vi "FindServo_NoWhile.vi"(0 "Amplitude Reference Array":refnum<vi>[](array[refnum]), 1 "Parameter Reference Arrary":refnum<vi>[](array[refnum]), 7 "Parameter Cluster":T1={"Αmplitude (Deg)"=0.0, "Amplitude (cm)"=4.0, "Frequency (Hz)"=1.0, "Number of Waves"=1.0, "Length of Segments (cm)"=10.0, "Wave Exponential"=2.0, "Number of Servos"=5.0, "Bend Amplitude 1"=0.1, "Bend Amplitude 2"=0.2, "Bend Phase 1"=0.0, "Bend Phase 2"=0.8499}, 8 "Wave Form":u16(ring) items=["Sine", "Exponentional Sine", "Two Beam Bending", "Flat Plate"], 12 "Wind Up":bool, 13 "Start Time (Tick Count-millis)":u32, 14 "Wind Down":bool, 15 "Wind Down Time":i32=5, 16 "Stop In":bool, 17 "Stop Pressed Shift In (False)":bool, 19 "Ms Since Stop Shift In (Start Time)":u32, 23 "Stop In Reference":refnum<vi>, 27 "S since stop Shift In":dbl) -> (18 "Stop Out":bool, 20 "phi":dbl[](array[numeric]), 21 "X Nodes":dbl[](array[numeric]), 22 "Y Nodes":dbl[](array[numeric]), 24 "Stop Pressed Shift Out (False)":bool, 25 "MS Since Stop Shift Out":u32, 26 "S since stop Shift Out":dbl)   [LabVIEW 2017]
panel:
  out "Simulation Time":dbl
  # "Off"
  # "On"
  # "Off"
  # "On"
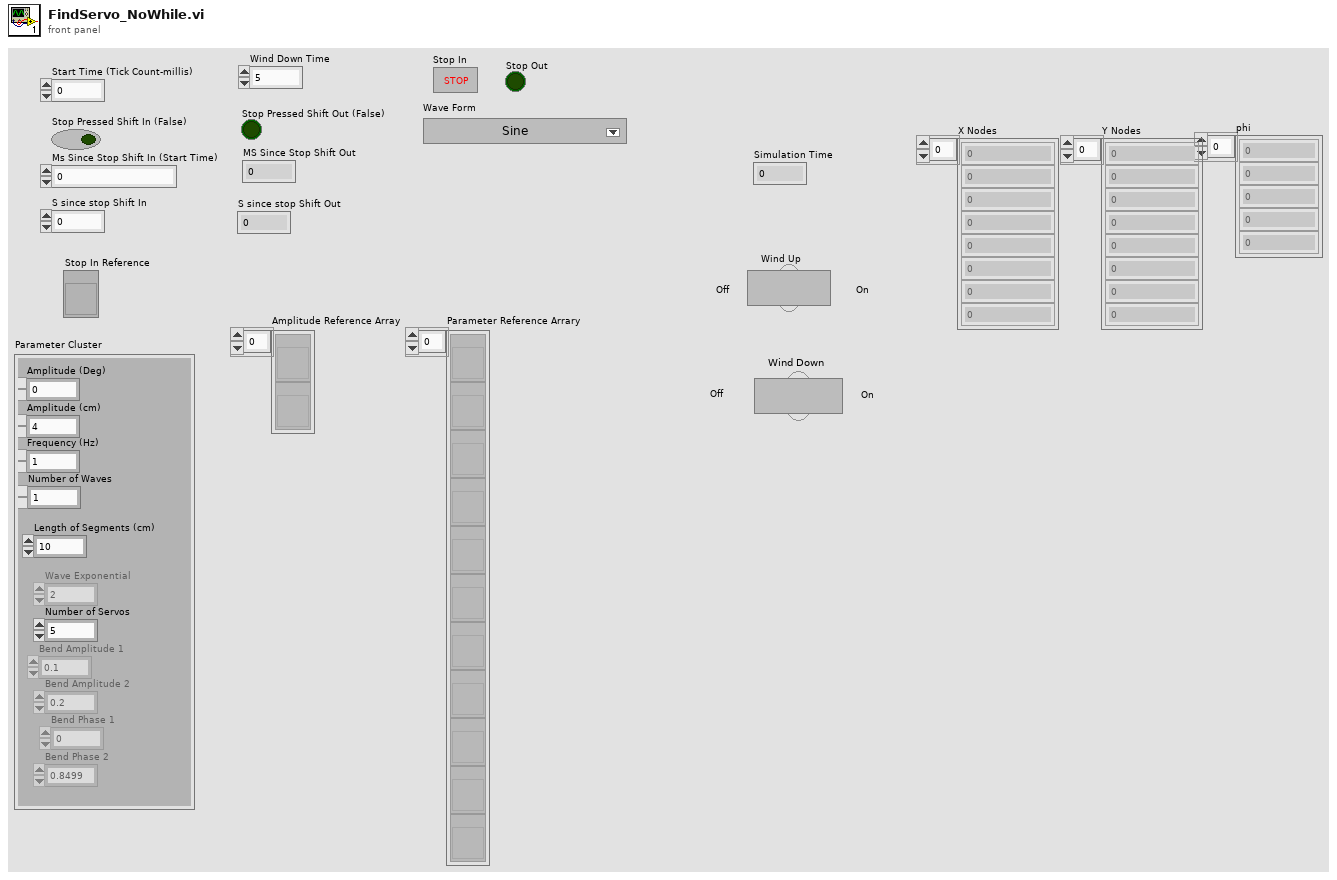
[diagram p1: front panel]
types:
  T1 = cluster{"Αmplitude (Deg)":dbl, "Amplitude (cm)":dbl, "Frequency (Hz)":dbl, "Number of Waves":dbl, "Length of Segments (cm)":dbl, "Wave Exponential":dbl, "Number of Servos":dbl, "Bend Amplitude 1":dbl, "Bend Amplitude 2":dbl, "Bend Phase 1":dbl, "Bend Phase 2":dbl}
  T2 = enum8{"Enabled", "Disabled", "Disabled and Grayed Out"}
  T3 = enum8{"Enabled", "Disabled", "Disabled and Grayed Out"}[]
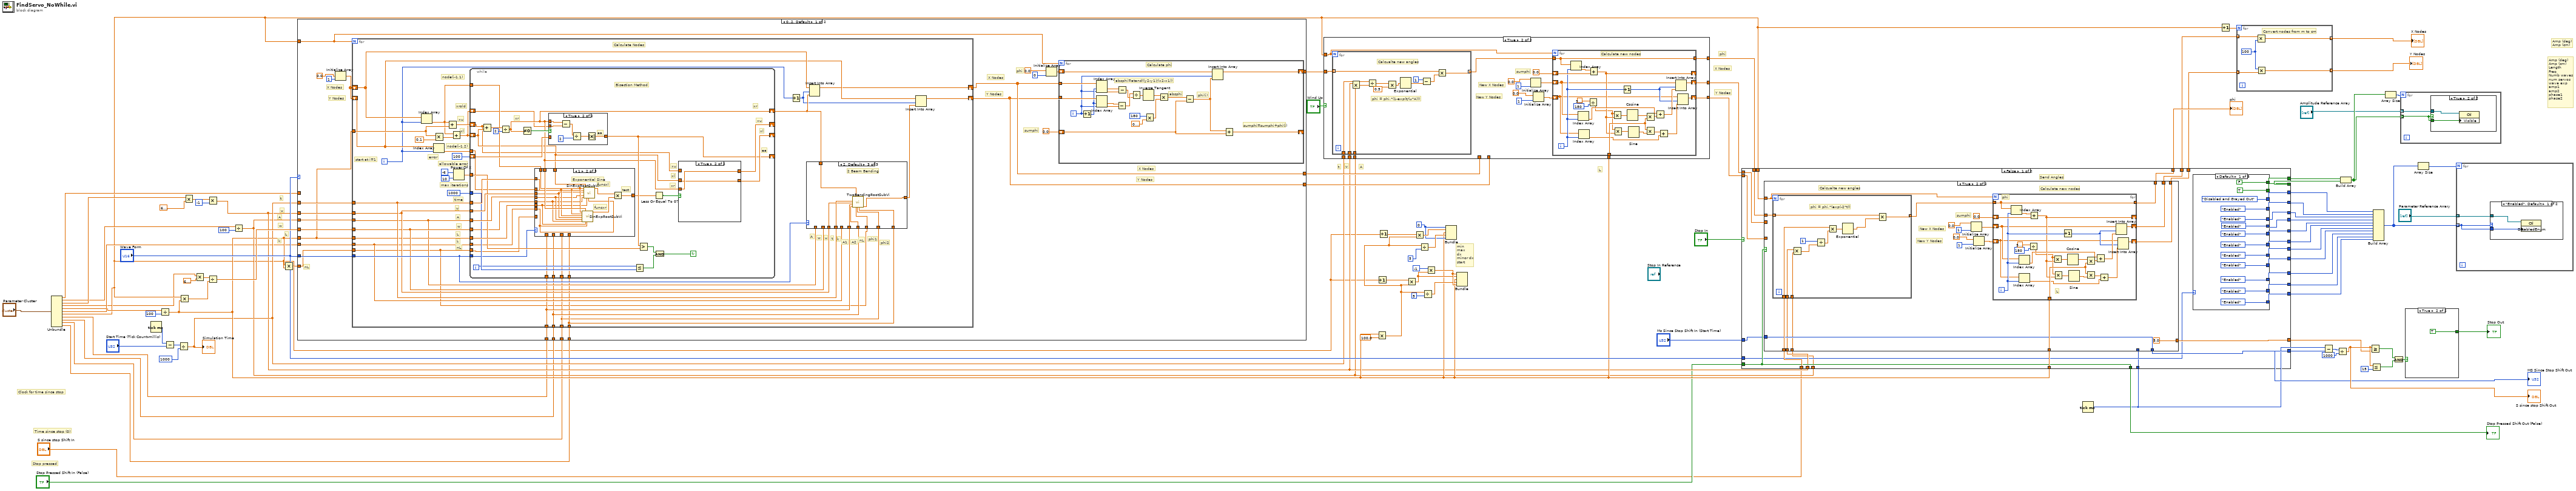
[diagram p0: block diagram]
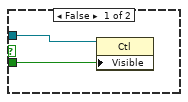
[diagram p2: hidden frame]
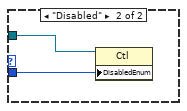
[diagram p3: hidden frame]
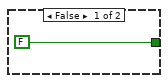
[diagram p4: hidden frame]
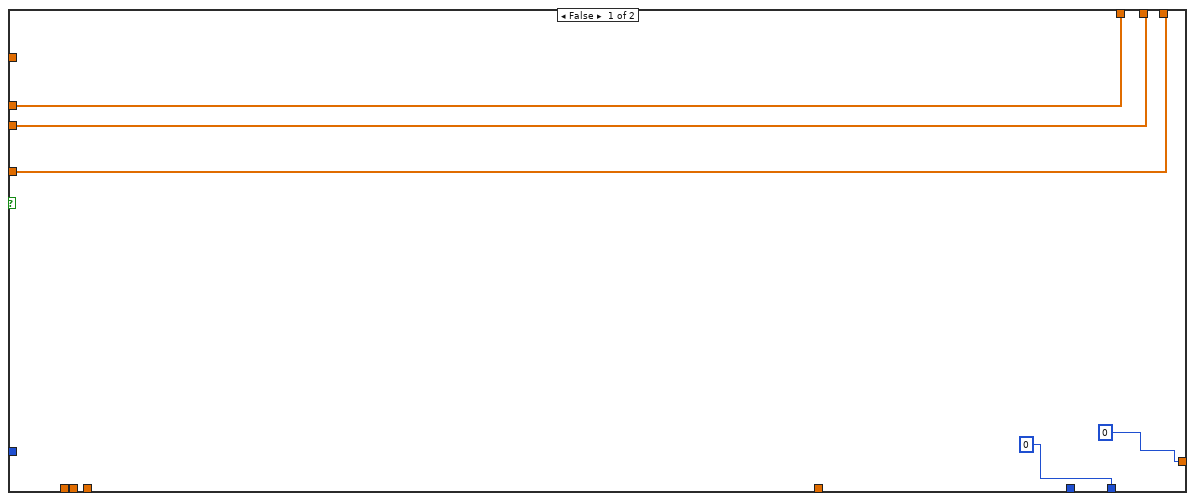
[diagram p5: hidden frame]
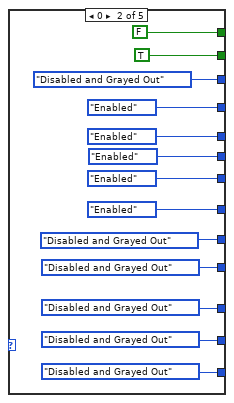
[diagram p6: hidden frame]
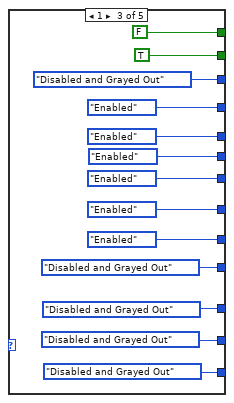
[diagram p7: hidden frame]
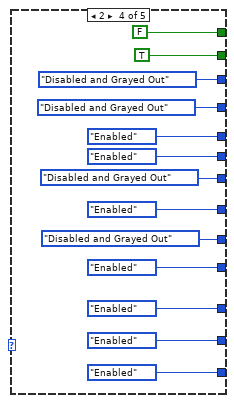
[diagram p8: hidden frame]
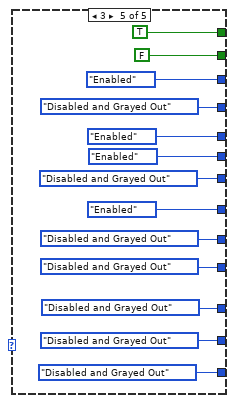
[diagram p9: hidden frame]
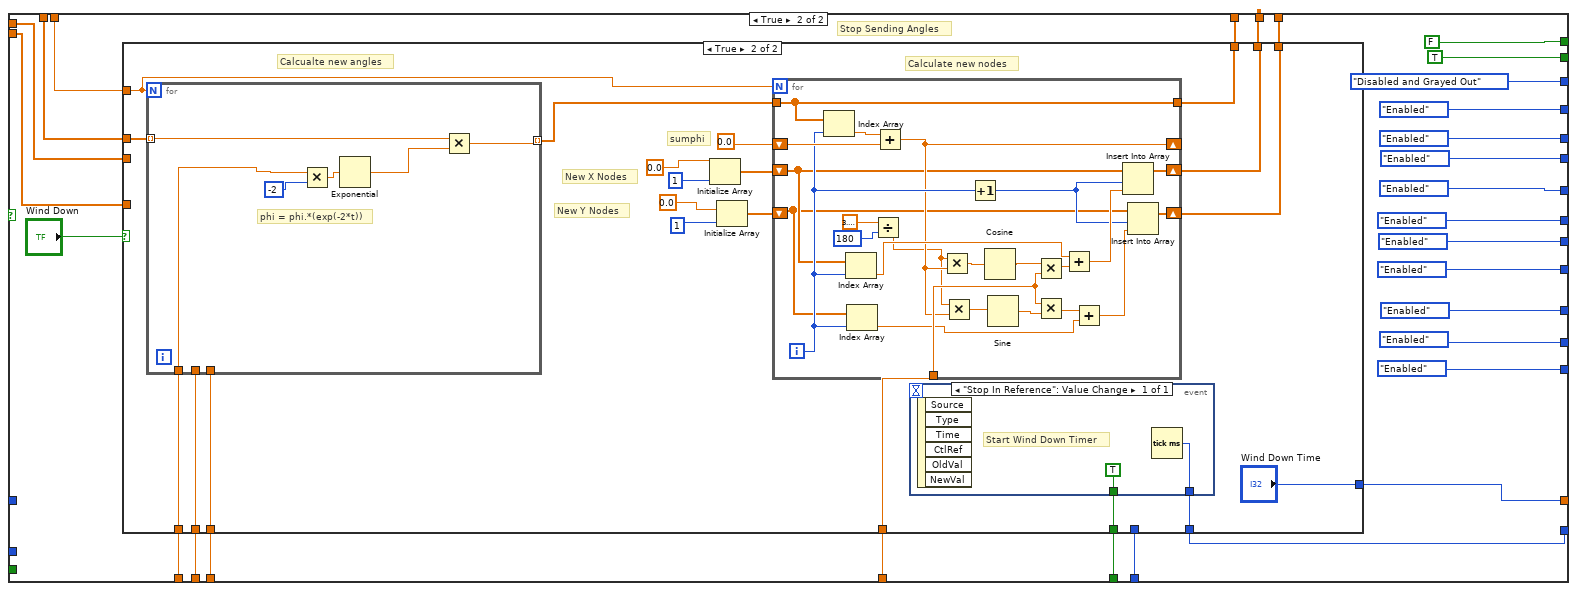
[diagram p10: hidden frame]
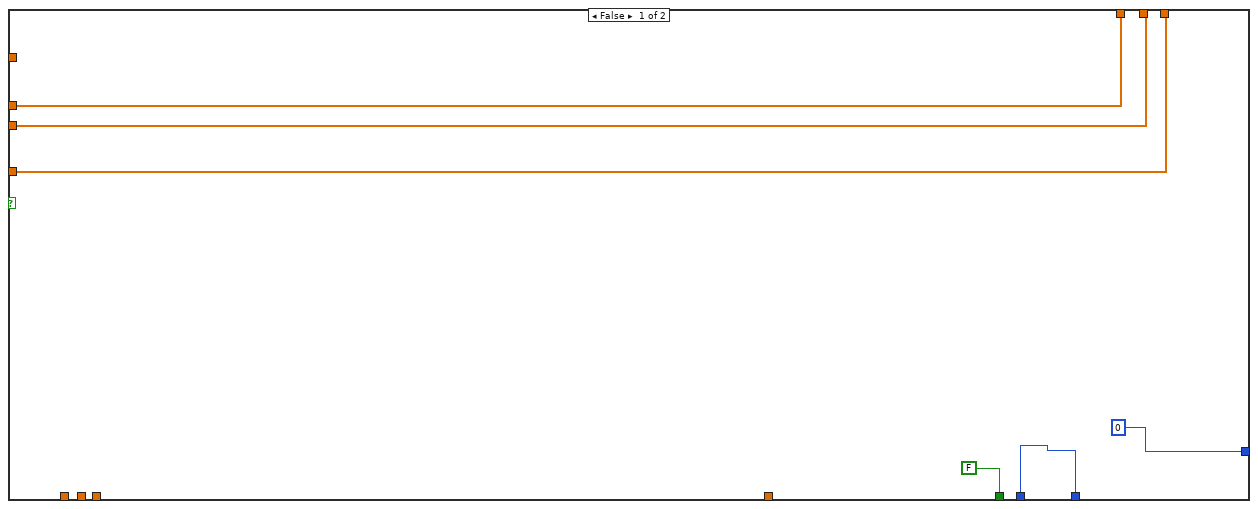
[diagram p11: hidden frame]
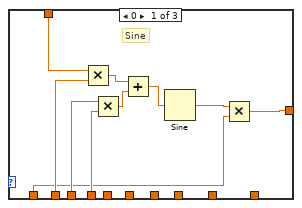
[diagram p12: hidden frame]
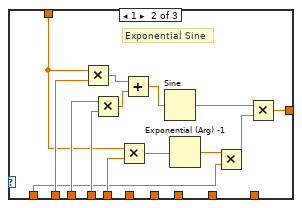
[diagram p13: hidden frame]
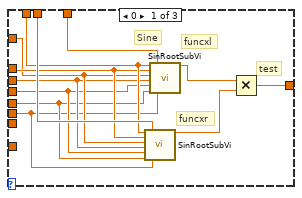
[diagram p16: hidden frame]
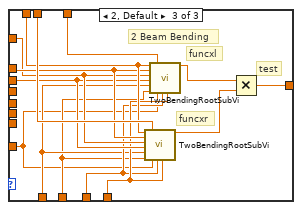
[diagram p17: hidden frame]
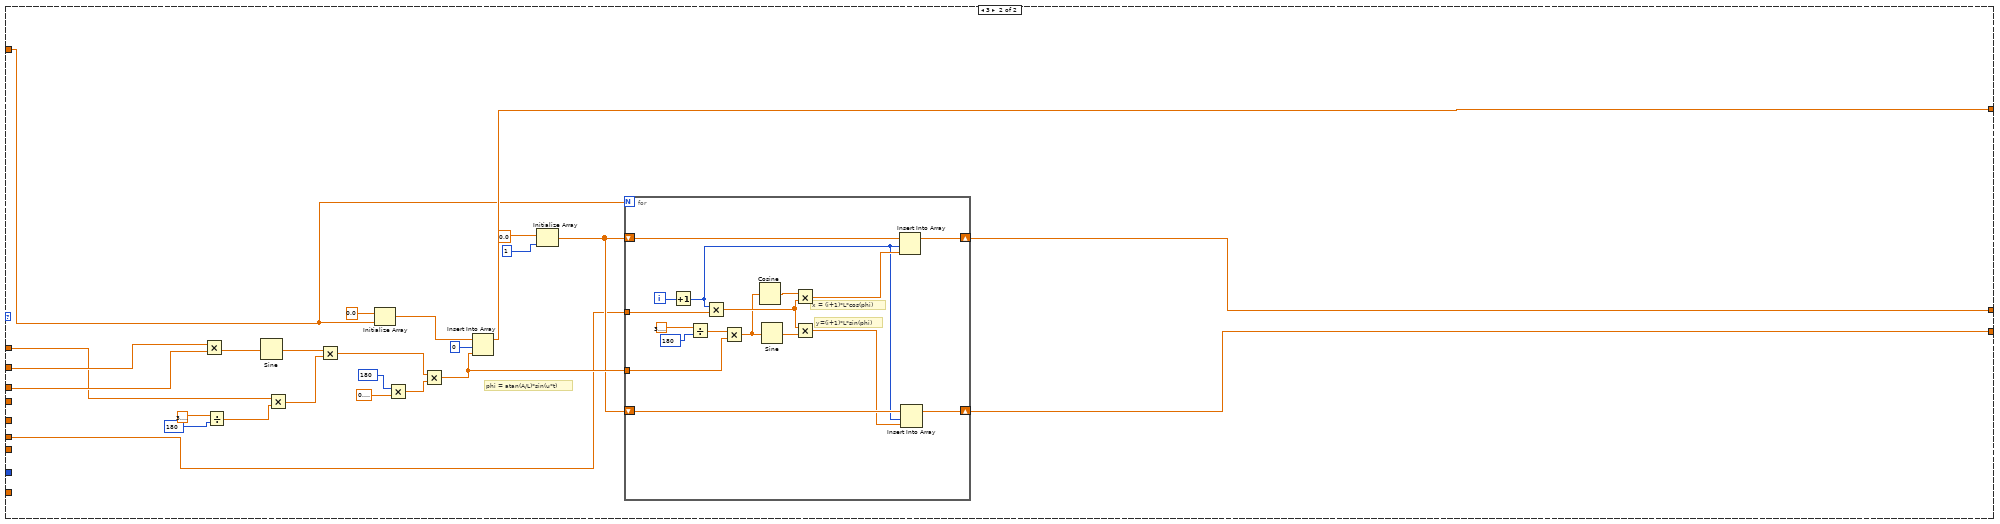
[diagram p18: hidden frame]
diagram:
  w65 = 0
  # "Amp (deg)\nAmp (cm)"
  # "Amp (deg)\nAmp (cm)\nLength\nFreq\nNumb waves\nnum servos\nwave exp\namp1\namp2\nphase1\nphase2"
  # "Y Nodes"
  # "X Nodes"
  # "phi"
  # "k"
  # "min\nmax\ndx\nminor dx\nstart"
  # "A"
  # "t"
  # "L"
  # "A"
  # "u"
  # "t"
  # "u"
  # "L"
  # "w"
  # "Stop pressed"
  # "Clock for time since stop"
  # "Time since stop (0)"
  n1 = Unbundle("Parameter Cluster") -> ("Αmplitude (Deg)"=w15:dbl, "Amplitude (cm)"=w13:dbl, "Frequency (Hz)"=w14:dbl, "Number of Waves"=w4:dbl, "Length of Segments (cm)"=w11:dbl, "Wave Exponential"=w12:dbl, "Number of Servos"=w5:dbl, "Bend Amplitude 1"=w6:dbl, "Bend Amplitude 2"=w10:dbl, "Bend Phase 1"=w9:dbl, "Bend Phase 2"=w8:dbl)
  n2 = Tick Count (ms)() -> (millisecond timer value=w81:u32)
  n3 = Divide(x=w11, y=100) -> (x/y=w59:dbl)
  n4 = Subtract(x=w81, y="Start Time (Tick Count-millis)") -> (x-y=w80:u32)
  n5 = Divide(x=w80, y=1000) -> (x/y=w58:dbl)
  "Simulation Time" <- w58
  n6 = Multiply(x=w5, y=w59) -> (x*y=w89:dbl)
  n7 = Multiply(x=w14, y=6.283185307179586) -> (x*y=w86:dbl)
  n8 = Multiply(x=w4, y=6.283185307179586) -> (x*y=w90:dbl)
  n9 = Multiply(x=w86, y=-1) -> (x*y=w57:dbl)
  n10 = Divide(x=w90, y=w89) -> (x/y=w84:dbl)
  n11 = Divide(x=w13, y=100) -> (x/y=w56:dbl)
  n12 = Multiply(x=w59, y=w5) -> (x*y=w62:dbl)
  n13 = case shown="0..2, Default" "Wave Form" {
    tunnel: "Wave Form" -> [w115 _]
    tunnel: w84 -> [w114 _]
    tunnel: [w110 w294] -> w82
    tunnel: w56 -> [w109 _]
    tunnel: w57 -> [w108 w308]
    tunnel: w58 -> [w107 w309]
    tunnel: w59 -> [w99 w291]
    tunnel: [w105 w293] -> w78
    tunnel: [w104 w292] -> w77
    tunnel: w5 -> [w103 w290]
    tunnel: w12 -> [w98 _]
    tunnel: w6 -> [w97 _]
    tunnel: w10 -> [w96 _]
    tunnel: w9 -> [w95 _]
    tunnel: w8 -> [w94 _]
    tunnel: w62 -> [w93 _]
    tunnel: w15 -> [_ w287]
    frame 0..2, Default {
      # "nL"
      # "Y Nodes"
      # "X Nodes"
      # "Y Nodes"
      # "X Nodes"
      # "Y Nodes"
      # "X Nodes"
      # "sumphi"
      # "phi"
      n14 = Initialize Array(0.0, 1) -> (w100:dbl[])
      n15 = for {
        N: w103 -> [_]
        shift-right: [w154] -> w105
        shift-left: w100 -> [w159]
        shift-right: [w153] -> w104
        shift-left: w100 -> [w158]
        tunnel: w99 -> [w167]
        tunnel: w107 -> [w151]
        tunnel: w108 -> [w150]
        tunnel: w109 -> [w143]
        tunnel: w114 -> [w149]
        tunnel: w99 -> [w148]
        tunnel: w115 -> [w157]
        tunnel: w98 -> [w142]
        tunnel: w97 -> [w141]
        tunnel: w96 -> [w140]
        tunnel: w95 -> [w138]
        tunnel: w94 -> [w139]
        tunnel: w93 -> [w137]
        i -> [w145]
        # "nL"
        # "phi2"
        # "phi1"
        # "nL"
        # "A2"
        # "A1"
        # "k"
        # "t"
        # "u"
        # "w"
        # "A"
        # "k"
        # "Calculate Nodes"
        # "xrold"
        # "error"
        # "L"
        # "w"
        # "A"
        # "u"
        # "time"
        # "allowable error"
        # "max iterations"
        # "node(i-1,2)"
        # "node(i-1,1)"
        # "xl"
        # "xu"
        # "start at i=1"
        n16 = Index Array(array=w159, index=w145) -> (element=w165:dbl)
        n17 = Index Array(array=w158, index=w145) -> (element=w164:dbl)
        n18 = Multiply(x=w167, y=0.1) -> (x*y=w166:dbl)
        n19 = Add(x=w165, y=w167) -> (x+y=w147:dbl)
        n20 = Add(x=w165, y=w166) -> (x+y=w146:dbl)
        n21 = Power Of X(1:10, 2:-6) -> (0:w156:dbl)
        n22 = while {
          tunnel: w165 -> [w215]
          tunnel: w164 -> [w214]
          tunnel: w156 -> [w226]
          tunnel: 1000 -> [w227]
          tunnel: w151 -> [w233]
          tunnel: w150 -> [w232]
          tunnel: w143 -> [w234]
          tunnel: w149 -> [w217]
          tunnel: w148 -> [w228]
          tunnel: w157 -> [w203]
          shift-right: [w216] -> w155
          shift-left: w146 -> [w213]
          shift-right: [w218] -> _
          shift-left: 100 -> [w229]
          shift-right: [w220] -> _
          shift-left: w147 -> [w211]
          shift-right: [w219] -> _
          shift-left: w146 -> [w212]
          tunnel: w142 -> [w208]
          tunnel: w141 -> [w207]
          tunnel: w140 -> [w206]
          tunnel: w138 -> [w205]
          tunnel: w139 -> [w204]
          tunnel: w137 -> [w202]
          i -> [w221]
          stop <- w223 continue-if-true
          # "Bisection Method"
          # "ea"
          # "xr"
          # "xu"
          # "xr"
          # "xl"
          # "xl"
          # "xu"
          # "xr"
          n23 = Add(x=w211, y=w212) -> (x+y=w231:dbl)
          n24 = Divide(x=w231, y=2) -> (x/y=w216:dbl)
          n25 = Not Equal To 0?(x=w216) -> (x != 0?=w225:bool)
          n26 = case shown="1" w203 {
            tunnel: w228 -> [w249 w262 _]
            tunnel: w217 -> [w250 w263 _]
            tunnel: w234 -> [w251 w264 _]
            tunnel: w232 -> [w252 w265 w279]
            tunnel: w233 -> [w253 w266 w280]
            tunnel: w214 -> [w254 w267 w281]
            tunnel: w215 -> [w255 w268 w282]
            tunnel: w212 -> [w257 w270 w284]
            tunnel: w216 -> [w256 w269 w283]
            tunnel: [w248 w260 w276] -> w209
            tunnel: w208 -> [_ w258 _]
            tunnel: w207 -> [_ _ w273]
            tunnel: w206 -> [_ _ w272]
            tunnel: w205 -> [_ _ w274]
            tunnel: w204 -> [_ _ w275]
            tunnel: w202 -> [_ _ w271]
            frame 0 {
              # "Sine"
              # "test"
              # "funcxr"
              # "funcxl"
              n27 = call "SinRootSubVi.vi"("x node"=w255, "y node"=w254, "time"=w253, "u"=w252, "A"=w251, "w"=w250, "x"=w256, "L"=w249) -> ("SinRoot"=w247:dbl)  [unwired: 9 in, 2 out]
              n28 = call "SinRootSubVi.vi"("x node"=w255, "y node"=w254, "time"=w253, "u"=w252, "A"=w251, "w"=w250, "x"=w257, "L"=w249) -> ("SinRoot"=w246:dbl)  [unwired: 9 in, 2 out]
              n29 = Multiply(x=w246, y=w247) -> (x*y=w248:dbl)
            }
            frame 1 {
              # "Exponential Sine"
              # "test"
              # "funcxr"
              # "funcxl"
              n30 = call "SinExpRootSubVi.vi"("x node"=w268, "y node"=w267, "time"=w266, "u"=w265, "A"=w264, "w"=w263, "x"=w269, "L"=w262, "k"=w258) -> ("SinExpRoot"=w261:dbl)  [unwired: 10 in]
              n31 = call "SinExpRootSubVi.vi"("x node"=w268, "y node"=w266, "time"=w265, "u"=w270, "A"=w264, "w"=w263, "x"=w267, "L"=w262, "k"=w258) -> ("SinExpRoot"=w259:dbl)  [unwired: 10 in]
              n32 = Multiply(x=w259, y=w261) -> (x*y=w260:dbl)
            }
            frame 2, Default {
              # "2 Beam Bending"
              # "test"
              # "funcxr"
              # "funcxl"
              n33 = call "TwoBendingRootSubVi.vi"("x node"=w282, "y node"=w281, "t"=w280, "u"=w279, "amp 1"=w273, "amp 2"=w272, "x"=w283, "nL"=w271, "phi 1"=w274, "phi 2"=w275) -> ("BendRoot"=w277:dbl)  [unwired: 8 in, 1 out]
              n34 = call "TwoBendingRootSubVi.vi"("x node"=w282, "y node"=w281, "t"=w280, "u"=w279, "amp 1"=w273, "amp 2"=w272, "x"=w284, "nL"=w271, "phi 1"=w274, "phi 2"=w275) -> ("BendRoot"=w278:dbl)  [unwired: 8 in, 1 out]
              n35 = Multiply(x=w278, y=w277) -> (x*y=w276:dbl)
            }
          }
          n36 = case shown="True" w225 {
            tunnel: w229 -> [w239 _]
            tunnel: w216 -> [_ w245]
            tunnel: w213 -> [_ w244]
            tunnel: [w239 w240] -> w218
            frame False {
            }
            frame True {
              # "ea"
              n37 = Subtract(x=w245, y=w244) -> (x-y=w242:dbl)
              n38 = Divide(x=w242, y=2) -> (x/y=w241:dbl)
              n39 = Absolute Value(x=w241) -> (abs(x)=w240:dbl)
            }
          }
          n40 = Less Or Equal?(x=w221, y=w227) -> (x <= y?=w224:bool)
          n41 = Greater?(x=w218, y=w226) -> (0:w222:bool)
          n42 = Less Or Equal To 0?(x=w209) -> (x <= 0?=w210:bool)
          n43 = And(x=w222, y=w224) -> (x .and. y?=w223:bool)
          n44 = case shown="True" w210 {
            tunnel: w212 -> [_ w237]
            tunnel: w216 -> [w235 w238]
            tunnel: w211 -> [w236 _]
            tunnel: [w236 w238] -> w220
            tunnel: [w235 w237] -> w219
            frame False {
            }
            frame True {
            }
          }
        }
        n45 = Increment(x=w145) -> (x+1=w144:i32)
        n46 = case shown="2, Default" w157 {
          tunnel: [w169 w185 w201] -> w152
          tunnel: w143 -> [w170 w180 _]
          tunnel: w149 -> [w175 w190 _]
          tunnel: w150 -> [w174 w189 w198]
          tunnel: w151 -> [w173 w188 w199]
          tunnel: w155 -> [w176 w184 w200]
          tunnel: w142 -> [_ w183 _]
          tunnel: w141 -> [_ _ w197]
          tunnel: w140 -> [_ _ w193]
          tunnel: w137 -> [_ _ w196]
          tunnel: w138 -> [_ _ w195]
          tunnel: w139 -> [_ _ w194]
          frame 0 {
            # "Sine"
            n47 = Multiply(x=w176, y=w175) -> (x*y=w178:dbl)
            n48 = Multiply(x=w174, y=w173) -> (x*y=w177:dbl)
            n49 = Add(x=w178, y=w177) -> (x+y=w172:dbl)
            n50 = Sine(x=w172) -> (sin(x)=w171:dbl)
            n51 = Multiply(x=w171, y=w170) -> (x*y=w169:dbl)
          }
          frame 1 {
            # "Exponential Sine"
            n52 = Multiply(x=w184, y=w190) -> (x*y=w192:dbl)
            n53 = Multiply(x=w189, y=w188) -> (x*y=w191:dbl)
            n54 = Multiply(x=w184, y=w183) -> (x*y=w182:dbl)
            n55 = Add(x=w192, y=w191) -> (x+y=w187:dbl)
            n56 = Sine(x=w187) -> (sin(x)=w186:dbl)
            n57 = Exponential (Arg) -1(1:w182) -> (0:w181:dbl)
            n58 = Multiply(x=w181, y=w180) -> (x*y=w179:dbl)
            n59 = Multiply(x=w186, y=w179) -> (x*y=w185:dbl)
          }
          frame 2, Default {
            # "2 Beam Bending"
            n60 = call "TwoBendingRootSubVi.vi"("t"=w199, "u"=w198, "amp 1"=w197, "amp 2"=w193, "x"=w200, "nL"=w196, "phi 1"=w195, "phi 2"=w194) -> ("Bend"=w201:dbl)  [unwired: 10 in, 1 out]
          }
        }
        n61 = Insert Into Array(array=w159, index=w144, new element=w155) -> (w154:dbl[])
        n62 = Insert Into Array(array=w158, index=w144, new element=w152) -> (w153:dbl[])
      }
      n63 = Initialize Array(0.0 ("element"), 0 ("dimension size")) -> (w111:dbl[])
      n64 = for {
        N: w103 -> [_]
        tunnel: w105 -> [w124]
        tunnel: w104 -> [w136]
        shift-right: [w120] -> w110
        shift-left: w111 -> [w121]
        shift-right: [w116] -> _
        shift-left: 0.0 -> [w118]
        i -> [w122]
        # "Calculate phi"
        # "sumphi=sumphi+phi(i)"
        # "phi(i)"
        # "absphi"
        # "absphi=atand((y2-y1)/(x2-x1))"
        n65 = Increment(x=w122) -> (x+1=w123:i32)
        n66 = Index Array(array=w124, index #1=w123, index #2=w122) -> (element #1=w135:dbl, element #2=w134:dbl)
        n67 = Index Array(array=w136, index #1=w123, index #2=w122) -> (element #1=w128:dbl, element #2=w127:dbl)
        n68 = Subtract(x=w128, y=w127) -> (x-y=w133:dbl)
        n69 = Subtract(x=w135, y=w134) -> (x-y=w132:dbl)
        n70 = Divide(x=w133, y=w132) -> (x/y=w126:dbl)
        n71 = Inverse Tangent(1:w126) -> (0:w125:dbl)
        n72 = Multiply(x=180, y=0.3183098861837907) -> (x*y=w129:dbl)
        n73 = Multiply(x=w125, y=w129) -> (x*y=w119:dbl)
        n74 = Subtract(x=w119, y=w118) -> (x-y=w117:dbl)
        n75 = Insert Into Array(array=w121, index=w122, new element=w117) -> (w120:dbl[])
        n76 = Add(x=w117, y=w118) -> (x+y=w116:dbl)
      }
    }
    frame 3 {
      # "phi = atan(A/L)*sin(u*t)"
      n77 = Multiply(x=w309, y=w308) -> (x*y=w307:dbl)
      n78 = Divide(x=3.141592653589793, y=180) -> (x/y=w286:dbl)
      n79 = Sine(x=w307) -> (sin(x)=w306:dbl)
      n80 = Multiply(x=w287, y=w286) -> (x*y=w285:dbl)
      n81 = Multiply(x=w306, y=w285) -> (x*y=w300:dbl)
      n82 = Initialize Array(0.0, w290) -> (w304:dbl[])
      n83 = Multiply(x=180, y=0.3183098861837907) -> (x*y=w299:dbl)
      n84 = Multiply(x=w300, y=w299) -> (x*y=w298:dbl)
      n85 = Insert Into Array(array=w304, index=0, new element=w298) -> (w294:dbl[])
      n86 = Initialize Array(0.0 ("element"), 1 ("dimension size")) -> (w295:dbl[])
      n87 = for {
        N: w290 -> [_]
        tunnel: w291 -> [w322]
        tunnel: w298 -> [w318]
        shift-right: [w315] -> w293
        shift-left: w295 -> [w316]
        shift-right: [w312] -> w292
        shift-left: w295 -> [w313]
        i -> [w324]
        # "y=(i+1)*L*sin(phi)"
        # "x = (i+1)*L*cos(phi)"
        n88 = Increment(x=w324) -> (x+1=w310:i32)
        n89 = Divide(x=3.141592653589793, y=180) -> (x/y=w319:dbl)
        n90 = Multiply(x=w310, y=w322) -> (x*y=w321:dbl)
        n91 = Multiply(x=w319, y=w318) -> (x*y=w317:dbl)
        n92 = Cosine(x=w317) -> (cos(x)=w326:dbl)
        n93 = Sine(x=w317) -> (sin(x)=w325:dbl)
        n94 = Multiply(x=w326, y=w321) -> (x*y=w314:dbl)
        n95 = Multiply(x=w321, y=w325) -> (x*y=w311:dbl)
        n96 = Insert Into Array(array=w316, index=w310, new element=w314) -> (w315:dbl[])
        n97 = Insert Into Array(array=w313, index=w310, new element=w311) -> (w312:dbl[])
      }
    }
  }
  n98 = case shown="True" "Wind Up" {
    tunnel: w82 -> [w329 w346]
    tunnel: [w329 w342] -> w60
    tunnel: w5 -> [_ w338]
    tunnel: w56 -> [_ w345]
    tunnel: w57 -> [_ w344]
    tunnel: w58 -> [_ w343]
    tunnel: [w328 w337] -> w55
    tunnel: [w327 w336] -> w54
    tunnel: w59 -> [_ w340]
    tunnel: w78 -> [w328 _]
    tunnel: w77 -> [w327 _]
    frame False {
    }
    frame True {
      # "New X Nodes"
      # "New Y Nodes"
      # "sumphi"
      n99 = for {
        N: w338 -> [_]
        tunnel: w346 -> [w375] mode=indexing
        tunnel: [w374] -> w339 mode=indexing
        tunnel: w345 -> [w382]
        tunnel: w344 -> [w381]
        tunnel: w343 -> [w379]
        # "Calcualte new angles"
        # "phi = phi.*(1-exp(t/(u*A)))"
        n100 = Multiply(x=w381, y=w382) -> (x*y=w380:dbl)
        n101 = Divide(x=w379, y=w380) -> (x/y=w372:dbl)
        n102 = Multiply(x=w372, y=0.5) -> (x*y=w373:dbl)
        n103 = Exponential(1:w373) -> (0:w378:dbl)
        n104 = Subtract(x=1, y=w378) -> (x-y=w376:dbl)
        n105 = Multiply(x=w375, y=w376) -> (x*y=w374:dbl)
      }
      n106 = Initialize Array(0.0 ("element"), 1 ("dimension size")) -> (w331:dbl[])
      n107 = Initialize Array(0.0 ("element"), 1 ("dimension size")) -> (w330:dbl[])
      n108 = for {
        N: w338 -> [_]
        shift-right: [w350] -> _
        shift-left: 0.0 -> [w370]
        tunnel: w339 -> [w369]
        tunnel: [w369] -> w342
        tunnel: w340 -> [w367]
        shift-right: [w360] -> w337
        shift-left: w331 -> [w348]
        shift-right: [w359] -> w336
        shift-left: w330 -> [w347]
        i -> [w358]
        # "Calculate new nodes"
        n109 = Index Array(array=w369, index=w358) -> (element=w368:dbl)
        n110 = Index Array(array=w348, index=w358) -> (element=w366:dbl)
        n111 = Index Array(array=w347, index=w358) -> (element=w363:dbl)
        n112 = Divide(x=3.141592653589793, y=180) -> (x/y=w349:dbl)
        n113 = Add(x=w368, y=w370) -> (x+y=w350:dbl)
        n114 = Multiply(x=w349, y=w350) -> (x*y=w352:dbl)
        n115 = Multiply(x=w349, y=w350) -> (x*y=w351:dbl)
        n116 = Increment(x=w358) -> (x+1=w357:i32)
        n117 = Cosine(x=w352) -> (cos(x)=w356:dbl)
        n118 = Sine(x=w351) -> (sin(x)=w355:dbl)
        n119 = Multiply(x=w356, y=w367) -> (x*y=w365:dbl)
        n120 = Multiply(x=w367, y=w355) -> (x*y=w364:dbl)
        n121 = Add(x=w366, y=w365) -> (x+y=w362:dbl)
        n122 = Add(x=w364, y=w363) -> (x+y=w361:dbl)
        n123 = Insert Into Array(array=w348, index=w357, new element=w362) -> (w360:dbl[])
        n124 = Insert Into Array(array=w347, index=w357, new element=w361) -> (w359:dbl[])
      }
    }
  }
  n125 = Multiply(x=w59, y=100.0) -> (x*y=w63:dbl)
  n126 = Increment(x=w5) -> (x+1=w75:dbl)
  n127 = Increment(x=w5) -> (x+1=w72:dbl)
  n128 = Multiply(x=w75, y=w63) -> (x*y=w73:dbl)
  n129 = Multiply(x=w72, y=w63) -> (x*y=w69:dbl)
  n130 = Divide(x=w63, y=5) -> (x/y=w70:dbl)
  n131 = Divide(x=w63, y=5) -> (x/y=w71:dbl)
  n132 = Multiply(x=-1, y=w73) -> (x*y=w74:dbl)
  n133 = Bundle(w65, w69, w59, w70, w65) -> ()  [unwired: 1 in, 1 out]
  n134 = Bundle(w74, w73, w59, w71, w74) -> ()  [unwired: 1 in, 1 out]
  n135 = Tick Count (ms)() -> (millisecond timer value=w41:u32)
  n136 = case shown="False" "Stop In" {
    tunnel: "Wave Form" -> [w386 _]
    tunnel: [w412 FALSE] -> w33
    tunnel: [w411 TRUE] -> w32
    tunnel: [w410 T2."Enabled" ("Disabled")] -> w19
    tunnel: [w409 T2."Enabled" ("Disabled")] -> w30
    tunnel: [w400 T2."Enabled" ("Disabled")] -> w29
    tunnel: [w408 T2."Disabled and Grayed Out" ("Disabled")] -> w31
    tunnel: [w407 T2."Enabled" ("Disabled")] -> w28
    tunnel: [w406 T2."Enabled" ("Disabled")] -> w27
    tunnel: [w405 T2."Enabled" ("Disabled")] -> w26
    tunnel: [w404 T2."Enabled" ("Disabled")] -> w25
    tunnel: [w403 T2."Enabled" ("Disabled")] -> w24
    tunnel: [w402 T2."Enabled" ("Disabled")] -> w23
    tunnel: [w401 T2."Enabled" ("Disabled")] -> w22
    tunnel: w5 -> [w397 w550]
    tunnel: w60 -> [w394 w549]
    tunnel: w59 -> [w399 w548]
    tunnel: "S since stop Shift In" -> [w398 w547]
    tunnel: w57 -> [w387 w546]
    tunnel: w56 -> [w385 w545]
    tunnel: w55 -> [w393 w544]
    tunnel: w54 -> [w392 w543]
    tunnel: [w383 w540] -> w53
    tunnel: [w395 w539] -> w52
    tunnel: [w396 w538] -> w35
    tunnel: "Stop Pressed Shift In (False)" -> [w391 _]
    tunnel: [w391 w542] -> w47
    tunnel: [w388 w541] -> w46
    tunnel: "Ms Since Stop Shift In (Start Time)" -> [w390 _]
    tunnel: [w389 w537] -> w45
    tunnel: w41 -> [w384 w536]
    frame False {
      # "Send Angles"
      n137 = case shown="True" w391 {
        tunnel: w394 -> [w417 w436]
        tunnel: [w417 w434] -> w383
        tunnel: w397 -> [_ w430]
        tunnel: w398 -> [_ w435]
        tunnel: [w416 w429] -> w395
        tunnel: [w415 w428] -> w396
        tunnel: w399 -> [_ w432]
        tunnel: w393 -> [w416 _]
        tunnel: w392 -> [w415 _]
        tunnel: [0 w421] -> w388
        tunnel: w390 -> [_ w421]
        tunnel: [0 5.0] -> w389
        tunnel: w387 -> [_ w419]
        tunnel: w385 -> [_ w418]
        tunnel: w384 -> [_ _]
        frame False {
        }
        frame True {
          # "New X Nodes"
          # "New Y Nodes"
          # "sumphi"
          # "Calculate new nodes"
          # "Calcualte new angles"
          n138 = for {
            N: w430 -> [_]
            tunnel: w436 -> [w470] mode=indexing
            tunnel: [w469] -> w431 mode=indexing
            tunnel: w435 -> [w468]
            tunnel: w419 -> [w464]
            tunnel: w418 -> [w465]
            # "phi = phi.*(exp(-2*t))"
            n139 = Multiply(x=w464, y=w465) -> (x*y=w463:dbl)
            n140 = Divide(x=1, y=w463) -> (x/y=w461:dbl)
            n141 = Multiply(x=w468, y=w461) -> (x*y=w467:dbl)
            n142 = Exponential(1:w467) -> (0:w466:dbl)
            n143 = Multiply(x=w470, y=w466) -> (x*y=w469:dbl)
          }
          n144 = Initialize Array(0.0 ("element"), 1 ("dimension size")) -> (w423:dbl[])
          n145 = Initialize Array(0.0 ("element"), 1 ("dimension size")) -> (w422:dbl[])
          n146 = for {
            N: w430 -> [_]
            shift-right: [w440] -> _
            shift-left: 0.0 -> [w460]
            tunnel: w431 -> [w459]
            tunnel: [w459] -> w434
            tunnel: w432 -> [w457]
            shift-right: [w450] -> w429
            shift-left: w423 -> [w438]
            shift-right: [w449] -> w428
            shift-left: w422 -> [w437]
            i -> [w448]
            # "phi"
            # "L"
            n147 = Index Array(array=w459, index=w448) -> (element=w458:dbl)
            n148 = Index Array(array=w438, index=w448) -> (element=w456:dbl)
            n149 = Index Array(array=w437, index=w448) -> (element=w453:dbl)
            n150 = Divide(x=3.141592653589793, y=180) -> (x/y=w439:dbl)
            n151 = Add(x=w458, y=w460) -> (x+y=w440:dbl)
            n152 = Multiply(x=w439, y=w440) -> (x*y=w442:dbl)
            n153 = Multiply(x=w439, y=w440) -> (x*y=w441:dbl)
            n154 = Increment(x=w448) -> (x+1=w447:i32)
            n155 = Cosine(x=w442) -> (cos(x)=w446:dbl)
            n156 = Sine(x=w441) -> (sin(x)=w445:dbl)
            n157 = Multiply(x=w446, y=w457) -> (x*y=w455:dbl)
            n158 = Multiply(x=w457, y=w445) -> (x*y=w454:dbl)
            n159 = Add(x=w456, y=w455) -> (x+y=w452:dbl)
            n160 = Add(x=w454, y=w453) -> (x+y=w451:dbl)
            n161 = Insert Into Array(array=w438, index=w447, new element=w452) -> (w450:dbl[])
            n162 = Insert Into Array(array=w437, index=w447, new element=w451) -> (w449:dbl[])
          }
        }
      }
      n163 = case shown="Default" w386 {
        tunnel: [FALSE FALSE FALSE FALSE TRUE] -> w412
        tunnel: [TRUE TRUE TRUE TRUE FALSE] -> w411
        tunnel: [T2."Enabled" ("Disabled") T2."Enabled" ("Disabled") T2."Enabled" ("Disabled") T2."Disabled and Grayed Out" ("Disabled") T2."Disabled and Grayed Out" ("Disabled")] -> w410
        tunnel: [T2."Enabled" ("Disabled") T2."Enabled" ("Disabled") T2."Enabled" ("Disabled") T2."Enabled" ("Disabled") T2."Enabled" ("Disabled")] -> w409
        tunnel: [T2."Enabled" ("Disabled") T2."Enabled" ("Disabled") T2."Enabled" ("Disabled") T2."Enabled" ("Disabled") T2."Enabled" ("Disabled")] -> w400
        tunnel: [T2."Disabled and Grayed Out" ("Disabled") T2."Disabled and Grayed Out" ("Disabled") T2."Disabled and Grayed Out" ("Disabled") T2."Disabled and Grayed Out" ("Disabled") T2."Enabled" ("Disabled")] -> w408
        tunnel: [T2."Enabled" ("Disabled") T2."Enabled" ("Disabled") T2."Enabled" ("Disabled") T2."Disabled and Grayed Out" ("Disabled") T2."Disabled and Grayed Out" ("Disabled")] -> w407
        tunnel: [T2."Enabled" ("Disabled") T2."Enabled" ("Disabled") T2."Enabled" ("Disabled") T2."Enabled" ("Disabled") T2."Enabled" ("Disabled")] -> w406
        tunnel: [T2."Enabled" ("Disabled") T2."Disabled and Grayed Out" ("Disabled") T2."Enabled" ("Disabled") T2."Disabled and Grayed Out" ("Disabled") T2."Disabled and Grayed Out" ("Disabled")] -> w405
        tunnel: [T2."Enabled" ("Disabled") T2."Disabled and Grayed Out" ("Disabled") T2."Disabled and Grayed Out" ("Disabled") T2."Enabled" ("Disabled") T2."Disabled and Grayed Out" ("Disabled")] -> w404
        tunnel: [T2."Enabled" ("Disabled") T2."Disabled and Grayed Out" ("Disabled") T2."Disabled and Grayed Out" ("Disabled") T2."Enabled" ("Disabled") T2."Disabled and Grayed Out" ("Disabled")] -> w403
        tunnel: [T2."Enabled" ("Disabled") T2."Disabled and Grayed Out" ("Disabled") T2."Disabled and Grayed Out" ("Disabled") T2."Enabled" ("Disabled") T2."Disabled and Grayed Out" ("Disabled")] -> w402
        tunnel: [T2."Enabled" ("Disabled") T2."Disabled and Grayed Out" ("Disabled") T2."Disabled and Grayed Out" ("Disabled") T2."Enabled" ("Disabled") T2."Disabled and Grayed Out" ("Disabled")] -> w401
        frame Default {
        }
        frame 0 {
        }
        frame 1 {
        }
        frame 2 {
        }
        frame 3 {
        }
      }
    }
    frame True {
      # "Stop Sending Angles"
      n164 = case shown="True" "Wind Down" {
        tunnel: w549 -> [w570 w590]
        tunnel: [w570 w586] -> w540
        tunnel: w550 -> [_ w582]
        tunnel: w545 -> [_ w589]
        tunnel: w546 -> [_ w588]
        tunnel: w547 -> [_ w587]
        tunnel: [w569 w581] -> w539
        tunnel: [w568 w580] -> w538
        tunnel: w548 -> [_ w584]
        tunnel: w544 -> [w569 _]
        tunnel: w543 -> [w568 _]
        tunnel: [FALSE w573] -> w542
        tunnel: [0 "Wind Down Time"] -> w537
        tunnel: [w565 w572] -> w541
        tunnel: w536 -> [w565 _]
        frame False {
        }
        frame True {
          # "New X Nodes"
          # "New Y Nodes"
          # "sumphi"
          # "Calculate new nodes"
          # "Calcualte new angles"
          n165 = for {
            N: w582 -> [_]
            tunnel: w590 -> [w622] mode=indexing
            tunnel: [w621] -> w583 mode=indexing
            tunnel: w589 -> [_]
            tunnel: w588 -> [_]
            tunnel: w587 -> [w617]
            # "phi = phi.*(exp(-2*t))"
            n166 = Multiply(x=w617, y=-2) -> (x*y=w618:dbl)
            n167 = Exponential(1:w618) -> (0:w619:dbl)
            n168 = Multiply(x=w622, y=w619) -> (x*y=w621:dbl)
          }
          n169 = Initialize Array(0.0 ("element"), 1 ("dimension size")) -> (w575:dbl[])
          n170 = Initialize Array(0.0 ("element"), 1 ("dimension size")) -> (w574:dbl[])
          n171 = for {
            N: w582 -> [_]
            shift-right: [w596] -> _
            shift-left: 0.0 -> [w616]
            tunnel: w583 -> [w615]
            tunnel: [w615] -> w586
            tunnel: w584 -> [w613]
            shift-right: [w606] -> w581
            shift-left: w575 -> [w594]
            shift-right: [w605] -> w580
            shift-left: w574 -> [w593]
            i -> [w604]
            n172 = Index Array(array=w615, index=w604) -> (element=w614:dbl)
            n173 = Index Array(array=w594, index=w604) -> (element=w612:dbl)
            n174 = Index Array(array=w593, index=w604) -> (element=w609:dbl)
            n175 = Divide(x=3.141592653589793, y=180) -> (x/y=w595:dbl)
            n176 = Add(x=w614, y=w616) -> (x+y=w596:dbl)
            n177 = Multiply(x=w595, y=w596) -> (x*y=w598:dbl)
            n178 = Multiply(x=w595, y=w596) -> (x*y=w597:dbl)
            n179 = Increment(x=w604) -> (x+1=w603:i32)
            n180 = Cosine(x=w598) -> (cos(x)=w602:dbl)
            n181 = Sine(x=w597) -> (sin(x)=w601:dbl)
            n182 = Multiply(x=w602, y=w613) -> (x*y=w611:dbl)
            n183 = Multiply(x=w613, y=w601) -> (x*y=w610:dbl)
            n184 = Add(x=w612, y=w611) -> (x+y=w608:dbl)
            n185 = Add(x=w610, y=w609) -> (x+y=w607:dbl)
            n186 = Insert Into Array(array=w594, index=w603, new element=w608) -> (w606:dbl[])
            n187 = Insert Into Array(array=w593, index=w603, new element=w607) -> (w605:dbl[])
          }
          n188 = event shown="[0] \"Stop In Reference\": Value Change" {
            selector: _ -> [_]
            dyn-events: _ -> [_]
            timeout: _ -> [_]
            tunnel: [TRUE] -> w573
            tunnel: [w591] -> w572
            event "Stop In Reference": Value Change {
              # "Start Wind Down Timer"
              n189 = event-data() -> ()  [unwired: 1 in, 6 out]
              n190 = Tick Count (ms)() -> (millisecond timer value=w591:u32)
            }
          }
        }
      }
    }
  }
  "phi" <- w53
  "Stop Pressed Shift Out (False)" <- w47
  "MS Since Stop Shift Out" <- w46
  n191 = Increment(x=w5) -> (x+1=w76:dbl)
  n192 = for {
    N: w76 -> [_]
    tunnel: w52 -> [w627] mode=indexing
    tunnel: w35 -> [w625] mode=indexing
    tunnel: [w624] -> w36 mode=indexing
    tunnel: [w623] -> w34 mode=indexing
    w626 = 100
    # "Convert nodes from m to cm"
    n193 = Multiply(x=w627, y=w626) -> (x*y=w624:dbl)
    n194 = Multiply(x=w626, y=w625) -> (x*y=w623:dbl)
  }
  "X Nodes" <- w36
  "Y Nodes" <- w34
  n195 = Subtract(x=w41, y=w46) -> (x-y=w49:u32)
  n196 = Divide(x=w49, y=1000) -> (x/y=w48:dbl)
  "S since stop Shift Out" <- w48
  n197 = Build Array(w33, w32) -> (w17:bool[])
  n198 = Greater Or Equal?(x=w48, y=w45) -> (x >= y?=w43:bool)
  n199 = Less Or Equal?(x=w48, y=15) -> (x <= y?=w42:bool)
  n200 = Build Array(w31, w19, w30, w29, w28, w27, w26, w25, w24, w23, w22) -> (w20:T3)
  n201 = Array Size(array=w17) -> (size(s)=w18:i32)
  n202 = And(x=w43, y=w42) -> (x .and. y?=w44:bool)
  n203 = for {
    N: w18 -> [_]
    tunnel: w17 -> [w628] mode=indexing
    tunnel: "Amplitude Reference Array" -> [w629] mode=indexing
    n204 = case shown="True" w628 {
      tunnel: w629 -> [w630 w633]
      tunnel: w628 -> [w631 w632]
      frame False {
        n205 = property on="Property Node" class="Ctl"(reference=w630, "Visible"=w631) -> ()  [unwired: 1 in, 2 out]
      }
      frame True {
        n206 = property on="Property Node" class="Ctl"(reference=w633, "Visible"=w632) -> ()  [unwired: 1 in, 2 out]
      }
    }
  }
  n207 = case shown="True" w44 {
    tunnel: [FALSE TRUE] -> w40
    frame False {
    }
    frame True {
    }
  }
  "Stop Out" <- w40
  n208 = Array Size(array=w20) -> (size(s)=w21:i32)
  n209 = for {
    N: w21 -> [_]
    tunnel: w20 -> [w637] mode=indexing
    tunnel: "Parameter Reference Arrary" -> [w636] mode=indexing
    n210 = case shown="\"Enabled\", Default" w637 {
      tunnel: w637 -> [w639 w641]
      tunnel: w636 -> [w638 w640]
      frame "Enabled", Default {
        n211 = property on="Property Node" class="Ctl"(reference=w638, "DisabledEnum"=w639) -> ()  [unwired: 1 in, 2 out]
      }
      frame "Disabled" {
        n212 = property on="Property Node" class="Ctl"(reference=w640, "DisabledEnum"=w641) -> ()  [unwired: 1 in, 2 out]
      }
    }
  }
